vi "Rd Wr System Settings.vi"(8 "error in (no error)":errorcluster, 10 "Write? (F:Read)":bool, 11 "System Settings":T1) -> (0 "error out":errorcluster, 3 "System Settings out":T1)   [LabVIEW 2024]
uses:
  typedefs/CC cluster System Settings.ctl
  2e80df6d-94aa-46b9-8b94-ceea8c057880.vi
  659fb017-0e9f-42f9-b06e-930303f00cbc.vi
  <vilib>/JDP Science/JSONtext/Find Item.vi
  <vilib>/JDP Science/JSONtext/Next JSON Value.vi
  <vilib>/JDP Science/JSONtext/String Subset.vi
  <vilib>/JDP Science/JSONtext/Parsing/Advance past next JSON Value (inlined COPY).vi
  <vilib>/JDP Science/JSONtext/Parsing/Advance past whitespace.vi
  <vilib>/JDP Science/JSONtext/Parsing/Advance past String.vi
  <vilib>/JDP Science/JSONtext/Parsing/Advance past Number.vi
  <vilib>/JDP Science/JSONtext/Parsing/Advance past Line Ending.vi
  <vilib>/JDP Science/JSONtext/Parsing/Parse Full Path or Item Name.vi
  <vilib>/JDP Science/JSONtext/Parsing/Advance past Array.vi
  <vilib>/JDP Science/JSONtext/Parsing/Advance past Object.vi
  <vilib>/JDP Science/JSONtext/support/Error Cluster From Code.vi
  <vilib>/JDP Science/JSONtext/Offset/Find Item Locations by Path.vi
  <vilib>/JDP Science/JSONtext/JSON text to Variant.vi
  <vilib>/JDP Science/JSONtext/Variant to JSON Text.vi
  <vilib>/JDP Science/JSONtext/Set Item.vi
  <vilib>/JDP Science/JSONtext/LVClass Serializer/JSONtext LVClass Serializer.lvclass
  <vilib>/JDP Science/JSONtext/JSONtext.lvlib
panel:
  in  "Settings File":string="CC System Settings.json"
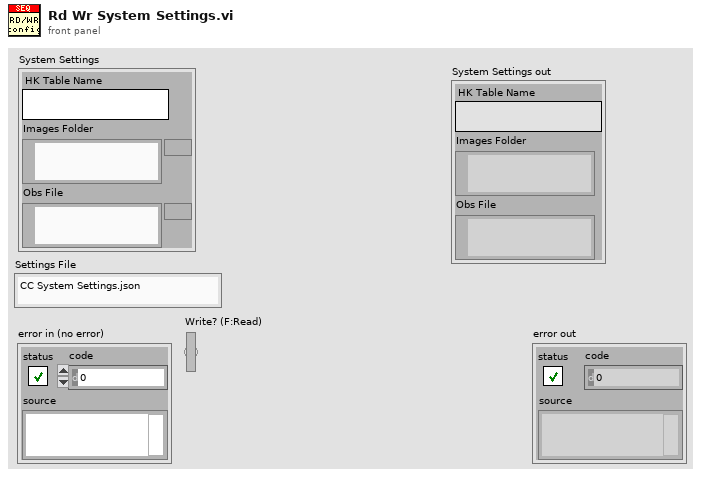
[diagram p1: front panel]
types:
  T1 = typedef "CC cluster System Settings.ctl" = cluster{"HK Table Name":string, "Images Folder":path, "Obs File":path}
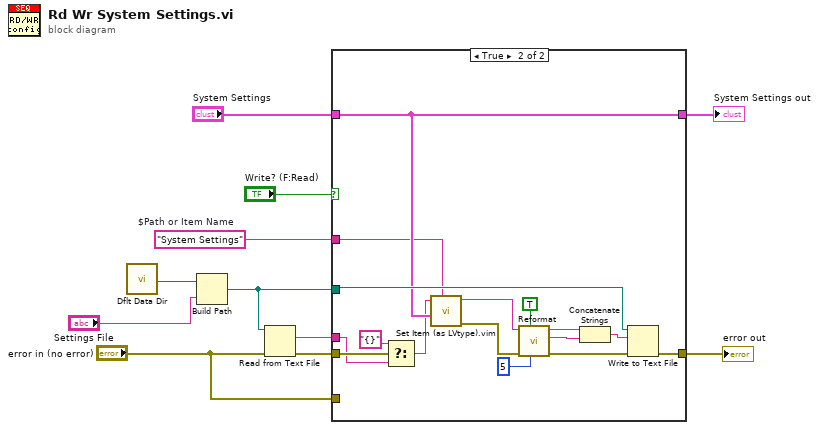
[diagram p0: block diagram]
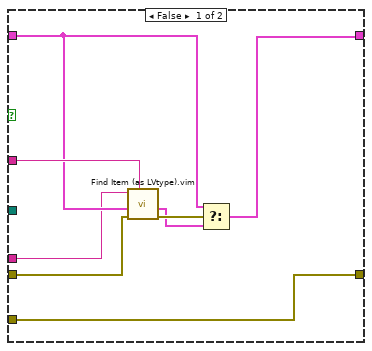
[diagram p2: hidden frame]
diagram:
  w5 = "System Settings"  # $Path or Item Name
  n1 = call <vilib>:"Dflt Data Dir.vi"() -> ("App:Default Data Directory"=w9:path)
  n2 = Build Path(base path=w9, name or relative path="Settings File") -> (appended path=w2:path)
  n3 = Read from Text File(file (use dialog)=w2, error in="error in (no error)") -> (text=w3:string, error out=w4:errorcluster)  [unwired: 2 in, 2 out]
  n4 = case shown="True" "Write? (F:Read)" {
    tunnel: w4 -> [w12 w31]
    tunnel: "System Settings" -> [w17 w33]
    tunnel: w2 -> [_ w35]
    tunnel: [w13 w34] -> w8
    tunnel: [w19 w33] -> w7
    tunnel: w5 -> [w18 w32]
    tunnel: w3 -> [w14 w29]
    tunnel: "error in (no error)" -> [w13 _]
    frame False {
      n5 = call "Find Item (as LVtype).vim"("$Path or Item Name"=w18, "error in (no error)"=w12, "Data Type and Default Value"=w17, "JSON"=w14) -> ("error out"=w16:errorcluster, "Data"=w15:T1)  [unwired: 4 in, 2 out]
      n6 = Select(t=w17, s=w16, f=w15) -> (s? t:f=w19:T1)
    }
    frame True {
      n7 = Select(t="{}" ("JSON"), s=w31, f=w29) -> (s? t:f=w28:string)
      n8 = call "Set Item (as LVtype).vim"("$Path or Item Name"=w32, "Anything"=w33, "JSON"=w28) -> ("error out"=w27:errorcluster, "<JSON>"=w22:string)  [unwired: 5 in, 1 out]
      n9 = call <vilib>:"Reformat.vi"("Pretty Print Levels"=5, "Alphabetically Sort Objects"=TRUE, "error in (no error)"=w27, "JSON"=w22) -> ("error out"=w26:errorcluster, "Rest of Input String"=w25:string, "<JSON>"=w20:string)  [unwired: 4 in, 1 out]
      n10 = Concatenate Strings(w20, w25) -> (w21:string)
      n11 = Write to Text File(file (use dialog)=w35, text=w21, error in=w26) -> (error out=w34:errorcluster)  [unwired: 1 in, 2 out]
    }
  }
  "error out" <- w8
  "System Settings out" <- w7
